vi "S2C_XML_SaveFile.vi"(8 "Error In":errorcluster) -> (0 "Error Out":errorcluster)   [LabVIEW 2015]
uses:
  S2C_XML_Globals.vi
  Globals/S2C_Globals.vi
  <resource>/objmgr/DOMUserDefRef.rc
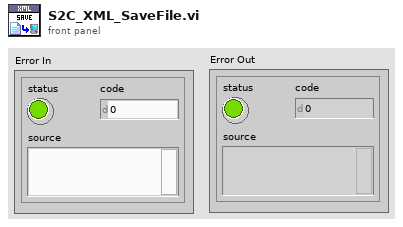
[diagram p1: front panel]
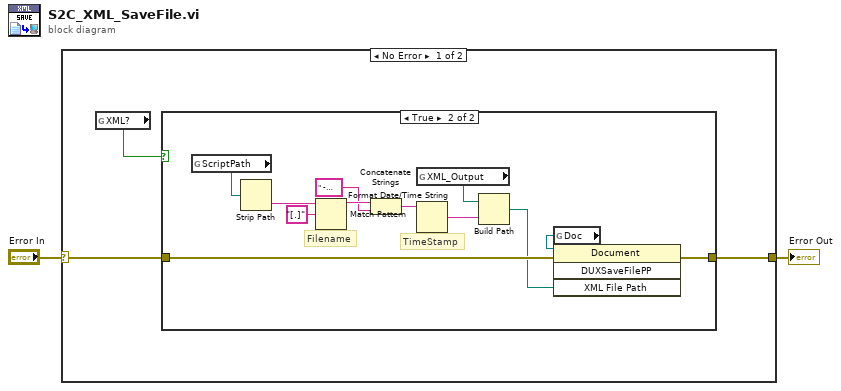
[diagram p0: block diagram]
diagram:
  n1 = case shown="No Error" "Error In" {
    selector: "Error In" -> [w5 w19]
    tunnel: [w4 w19] -> w1
    frame No Error {
      n2 = global read "S2C_XML_Globals.vi" "XML?"() -> (w3:bool)
      n3 = case shown="True" w3 {
        tunnel: w5 -> [w6 w9]
        tunnel: [w6 w8] -> w4
        frame False {
          # "The XML Output is currently disabled"
        }
        frame True {
          # "TimeStamp"
          # "Filename"
          n4 = global read "S2C_Globals.vi" "ScriptPath"() -> (w15:path)
          n5 = Strip Path(path=w15) -> (name=w16:string)  [unwired: 1 out]
          n6 = Match Pattern(string=w16, regular expression="[.]") -> (before substring=w14:string)  [unwired: 1 in, 3 out]
          n7 = Concatenate Strings(w14, " - [%m_%d_%Y - %I_%M_%S %p].xml" ("time format string (%c)")) -> (w13:string)
          n8 = global read "S2C_XML_Globals.vi" "XML_Output"() -> (w11:path)
          n9 = Format Date/Time String(time format string (%c)=w13) -> (date/time string=w18:string)  [unwired: 2 in]
          n10 = Build Path(base path=w11, name or relative path=w18) -> (appended path=w7:path)
          n11 = global read "S2C_XML_Globals.vi" "Doc"() -> (w10:refnum<k20>)
          n12 = invoke class="Document" method="DUXSaveFilePP"(reference=w10, error in=w9, "XML File Path"=w7) -> (error out=w8:errorcluster)  [unwired: 1 in, 3 out]
        }
      }
    }
    frame Error {
    }
  }
  "Error Out" <- w1
